vi "Device Info Dialog.vi"() -> ()   [LabVIEW 2011, in "CAN FD.lvlib"]
uses:
  CAN FD.lvlib
panel:
  in  "OK":bool
  out "type":string caption="硬件类型："
  out "SN":string caption="序列号："
  out "can_Num":u8 caption="CAN通道数："
  out "irq_Num":u16 caption="板卡中断号："
  out "in_ver":dbl caption="动态库版本：" format="%.2f"
  out "dr_ver":dbl caption="驱动版本：" format="%.2f"
  out "fw_ver":dbl caption="固件版本：" format="%.2f"
  out "hw_ver":dbl caption="硬件版本：" format="%.2f"
  # "硬件信息"
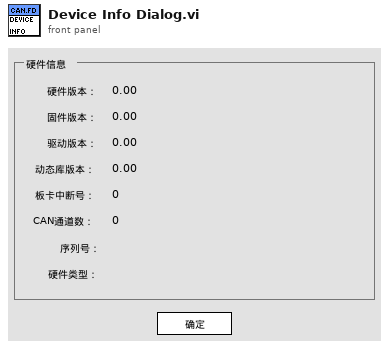
[diagram p1: front panel]
types:
  T1 = cluster{"hw_ver":dbl, "fw_ver":dbl, "dr_ver":dbl, "in_ver":dbl, "irq_Num":u16, "can_Num":u8, "SN":string, "hw_type":string}
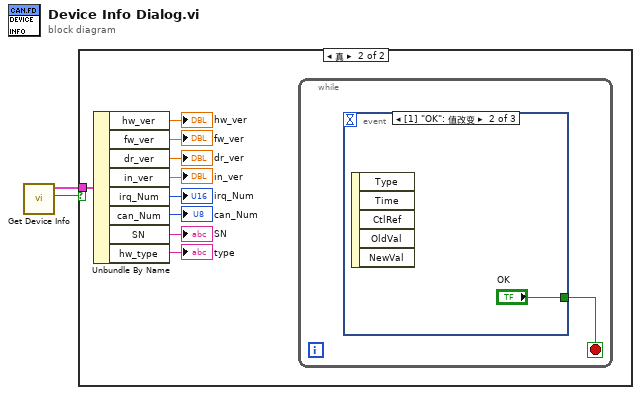
[diagram p0: block diagram]
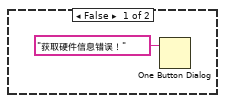
[diagram p2: hidden frame]
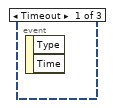
[diagram p3: hidden frame]
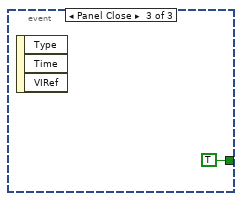
[diagram p4: hidden frame]
diagram:
  n1 = call "Get Device Info.vi"() -> ("Success"=w2:bool, "device info"=w1:T1)  [unwired: 9 in, 1 out]
  n2 = case shown="真" w2 {
    tunnel: w1 -> [_ w12]
    frame False {
      n3 = One Button Dialog(message="获取硬件信息错误！" ("消息")) -> ()  [unwired: 1 in, 1 out]
    }
    frame True {
      n4 = Unbundle By Name(w12) -> ("hw_ver"=→"hw_ver":dbl, "fw_ver"=→"fw_ver":dbl, "dr_ver"=→"dr_ver":dbl, "in_ver"=→"in_ver":dbl, "irq_Num"=→"irq_Num":u16, "can_Num"=→"can_Num":u8, "SN"=→"SN":string, "hw_type"=→"type":string)
      n5 = while {
        stop <- w13 stop-if-true
        n6 = event shown="[1] \"OK\": 值改变" {
          selector: _ -> [_ _ _]
          dyn-events: _ -> [_ _ _]
          timeout: _ -> [_ _ _]
          tunnel: [_ "OK" TRUE ("OK")] -> w13
          event Timeout {
            n7 = event-data() -> ()  [unwired: 1 in, 2 out]
          }
          event "OK": Value Change {
            n8 = event-data() -> ()  [unwired: 1 in, 5 out]
          }
          event Panel Close {
            n9 = event-data() -> ()  [unwired: 1 in, 3 out]
          }
        }
      }
    }
  }
